vi "Basic Auton.vi"(1 "Auton RPM":dbl=4200.0, 2 "Auton Pitch":dbl=30.5) -> ()   [LabVIEW 2012]
uses:
  Robot Global Data.vi
panel:
  in  "stop log":bool
  in  "System Data On?":bool=TRUE
  in  "Sample?":bool=TRUE
  in  "Sample Rate (sec)":dbl=0.03
  out "Prime 3":i32
  out "Report 2":i32
  out "S3":i32
  out "Count 3":bool
  out "Prime 2.1":i32
  out "Prime 2":i32
  out "Report 1":i32
  out "S2":i32
  out "Count 2":bool
  out "Prime 1.1":i32
  out "Prime 1":i32
  out "S1":i32
  out "Count 1":bool
  # "Pre-Shot"
  # "Shoot 1"
  # "Shoot 2"
  # "Shoot 3"
  # "Was 0.1 at Palmetto"
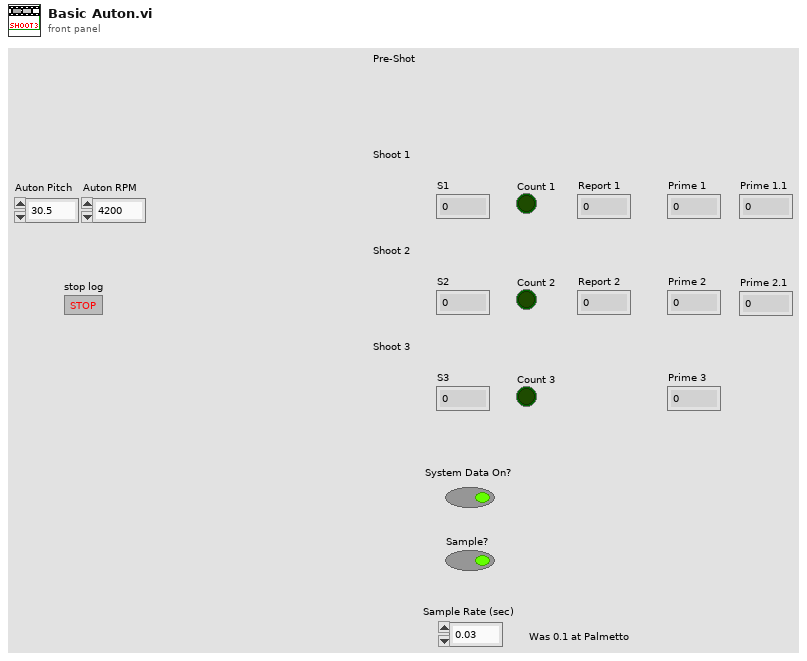
[diagram p1: front panel]
types:
  T1 = enum16{"open", "open or create", "create or replace", "create", "open (read-only)"}
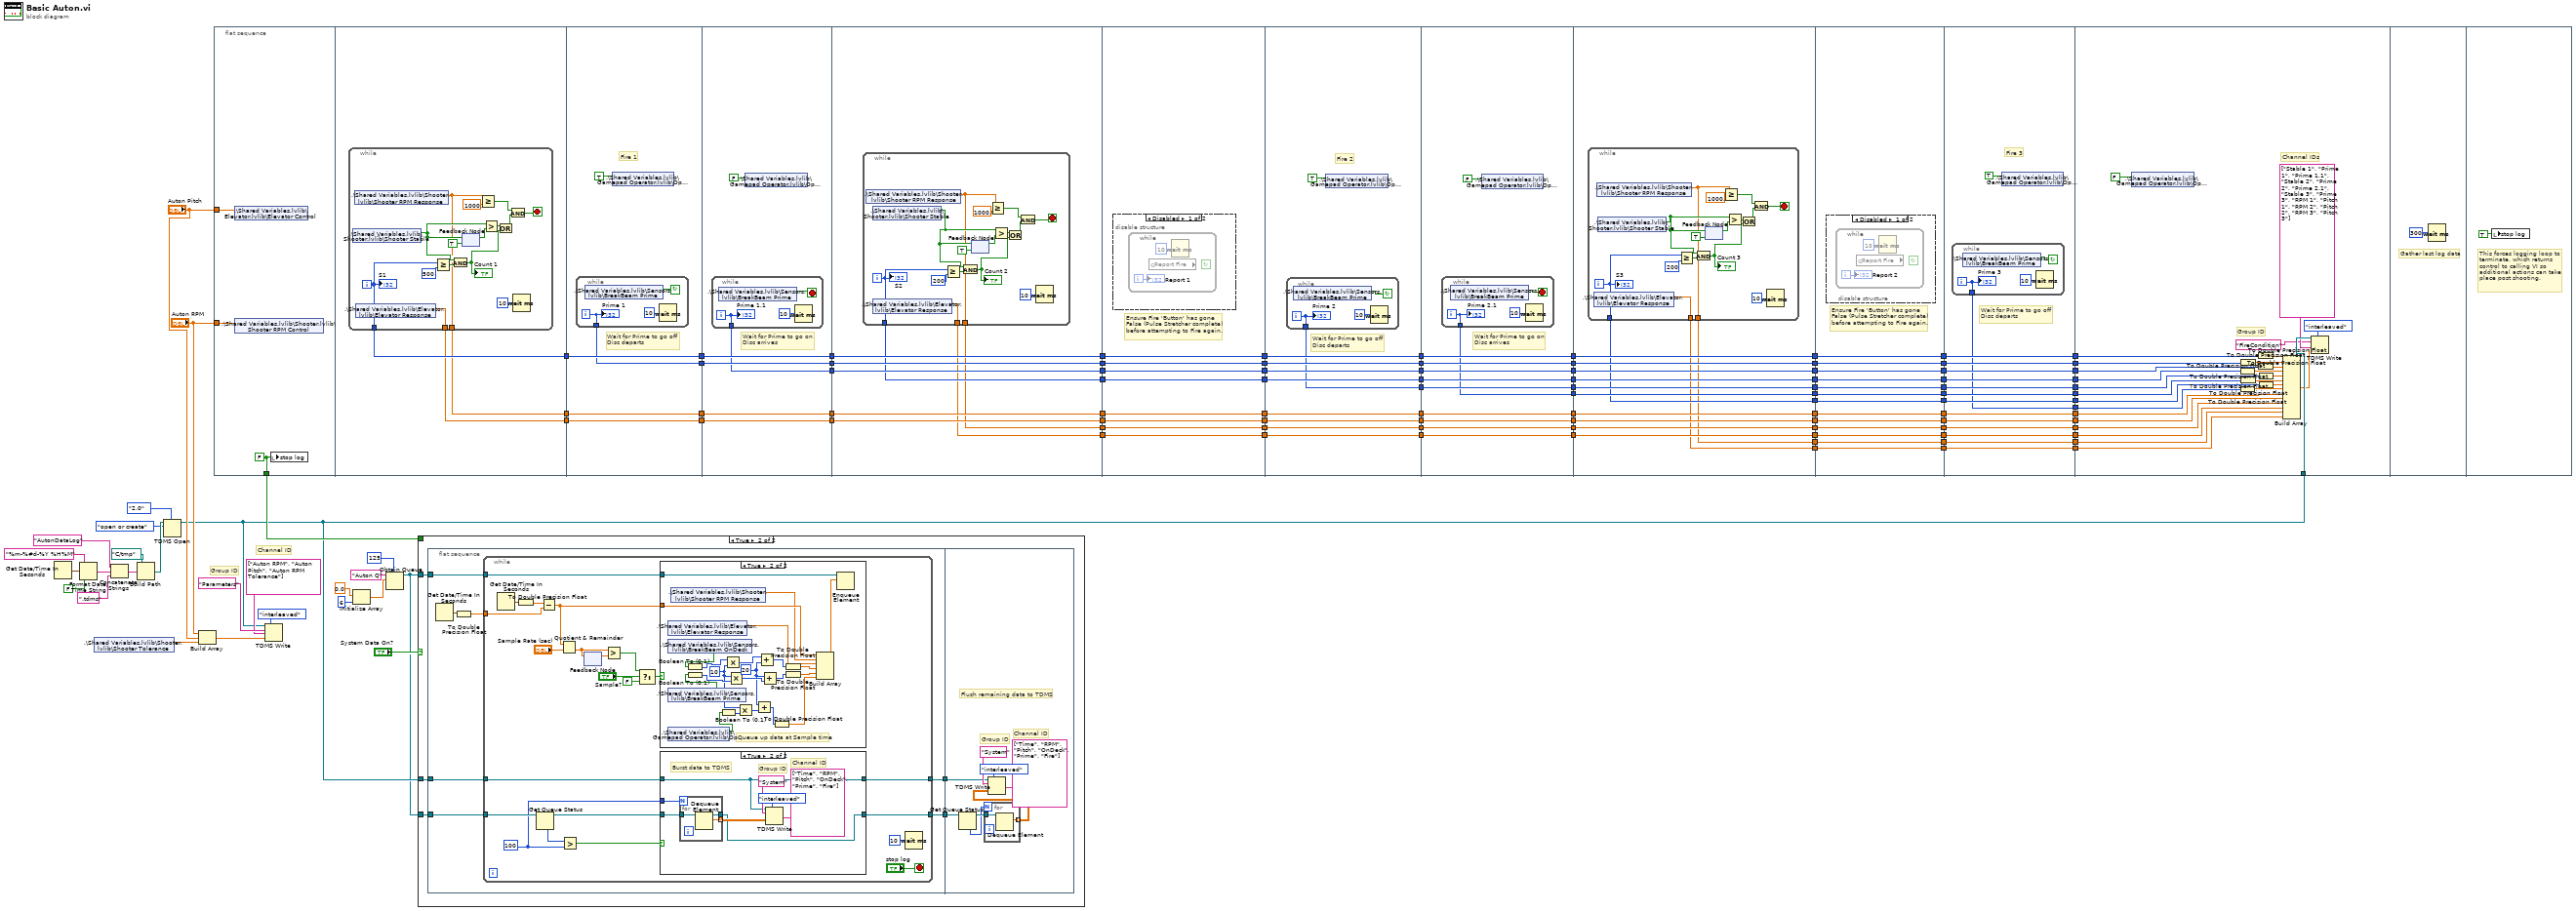
[diagram p0: block diagram]
diagram:
  # "Channel ID"
  # "Group ID"
  n1 = Get Date/Time In Seconds() -> (seconds since 1Jan1904=w17:timestamp)
  n2 = Format Date/Time String(time format string (%c)="%m-%#d-%Y %H%M", seconds (now)=w17, UTC format=FALSE) -> (date/time string=w22:string)
  n3 = shared-variable ".\\Shared Variables.lvlib\\Shooter.lvlib\\Shooter Tolerance"() -> (w10:dbl)  [unwired: 1 in, 1 out]
  n4 = Concatenate Strings("AutonDataLog" ("string"), w22, ".tdms" ("string")) -> (w24:string)
  n5 = Build Path(base path=path "C:/tmp" ("file path (dialog if empty)"), name or relative path=w24) -> (appended path=w25:path)
  n6 = TDMS Open(7:enum16{"1.0", "2.0"}."2.0" ("file format version (2.0)"), 10:T1."open or create" ("operation (0:open)"), 11:w25) -> (3:w7:refnum<k34>)  [unwired: 3 in, 1 out]
  n7 = Build Array("Auton RPM", "Auton Pitch", w10) -> (w13:dbl[])
  n8 = flat-sequence {
    tunnel: "Auton Pitch" -> [w116]
    tunnel: "Auton RPM" -> [w117]
    tunnel: [w115] -> w8
    tunnel: [w120] -> w114
    tunnel: [w119] -> w58
    tunnel: [w118] -> w48
    tunnel: w114 -> [w140]
    tunnel: [w140] -> w112
    tunnel: [w139] -> w96
    tunnel: [w138] -> w59
    tunnel: w58 -> [w138]
    tunnel: [w137] -> w49
    tunnel: w48 -> [w137]
    tunnel: [w149] -> w113
    tunnel: w112 -> [w149]
    tunnel: [w148] -> w97
    tunnel: w96 -> [w148]
    tunnel: [w147] -> w88
    tunnel: [w146] -> w60
    tunnel: w59 -> [w146]
    tunnel: [w145] -> w50
    tunnel: w49 -> [w145]
    tunnel: w113 -> [w160]
    tunnel: [w160] -> w108
    tunnel: [w159] -> w98
    tunnel: w97 -> [w159]
    tunnel: [w158] -> w89
    tunnel: w88 -> [w158]
    tunnel: [w157] -> w81
    tunnel: [w156] -> w61
    tunnel: w60 -> [w156]
    tunnel: [w155] -> w51
    tunnel: w50 -> [w155]
    tunnel: [w154] -> w41
    tunnel: [w153] -> w34
    tunnel: [w183] -> w109
    tunnel: w108 -> [w183]
    tunnel: [w182] -> w99
    tunnel: w98 -> [w182]
    tunnel: [w181] -> w90
    tunnel: w89 -> [w181]
    tunnel: [w180] -> w82
    tunnel: w81 -> [w180]
    tunnel: [w179] -> w62
    tunnel: w61 -> [w179]
    tunnel: [w178] -> w52
    tunnel: w51 -> [w178]
    tunnel: [w177] -> w42
    tunnel: w41 -> [w177]
    tunnel: [w176] -> w35
    tunnel: w34 -> [w176]
    tunnel: [w195] -> w110
    tunnel: w109 -> [w195]
    tunnel: [w194] -> w100
    tunnel: w99 -> [w194]
    tunnel: [w193] -> w91
    tunnel: w90 -> [w193]
    tunnel: [w192] -> w83
    tunnel: w82 -> [w192]
    tunnel: [w191] -> w76
    tunnel: [w190] -> w63
    tunnel: w62 -> [w190]
    tunnel: [w189] -> w53
    tunnel: w52 -> [w189]
    tunnel: [w188] -> w43
    tunnel: w42 -> [w188]
    tunnel: [w187] -> w36
    tunnel: w35 -> [w187]
    tunnel: [w209] -> w111
    tunnel: w110 -> [w209]
    tunnel: [w208] -> w101
    tunnel: w100 -> [w208]
    tunnel: [w207] -> w92
    tunnel: w91 -> [w207]
    tunnel: [w206] -> w84
    tunnel: w83 -> [w206]
    tunnel: [w205] -> w77
    tunnel: w76 -> [w205]
    tunnel: [w204] -> w72
    tunnel: [w203] -> w64
    tunnel: w63 -> [w203]
    tunnel: [w202] -> w54
    tunnel: w53 -> [w202]
    tunnel: [w201] -> w44
    tunnel: w43 -> [w201]
    tunnel: [w200] -> w37
    tunnel: w36 -> [w200]
    tunnel: w111 -> [w225]
    tunnel: [w225] -> w105
    tunnel: [w224] -> w102
    tunnel: w101 -> [w224]
    tunnel: [w223] -> w93
    tunnel: w92 -> [w223]
    tunnel: [w222] -> w85
    tunnel: w84 -> [w222]
    tunnel: [w221] -> w78
    tunnel: w77 -> [w221]
    tunnel: [w220] -> w73
    tunnel: w72 -> [w220]
    tunnel: [w219] -> w69
    tunnel: [w218] -> w65
    tunnel: w64 -> [w218]
    tunnel: [w217] -> w55
    tunnel: w54 -> [w217]
    tunnel: [w216] -> w45
    tunnel: w44 -> [w216]
    tunnel: [w215] -> w38
    tunnel: w37 -> [w215]
    tunnel: [w214] -> w31
    tunnel: [w213] -> w28
    tunnel: [w253] -> w106
    tunnel: w105 -> [w253]
    tunnel: [w252] -> w103
    tunnel: w102 -> [w252]
    tunnel: [w251] -> w94
    tunnel: w93 -> [w251]
    tunnel: [w250] -> w86
    tunnel: w85 -> [w250]
    tunnel: [w249] -> w79
    tunnel: w78 -> [w249]
    tunnel: [w248] -> w74
    tunnel: w73 -> [w248]
    tunnel: [w247] -> w70
    tunnel: w69 -> [w247]
    tunnel: [w246] -> w66
    tunnel: w65 -> [w246]
    tunnel: [w245] -> w56
    tunnel: w55 -> [w245]
    tunnel: [w244] -> w46
    tunnel: w45 -> [w244]
    tunnel: [w243] -> w39
    tunnel: w38 -> [w243]
    tunnel: [w242] -> w32
    tunnel: w31 -> [w242]
    tunnel: [w241] -> w29
    tunnel: w28 -> [w241]
    tunnel: [w270] -> w107
    tunnel: w106 -> [w270]
    tunnel: [w269] -> w104
    tunnel: w103 -> [w269]
    tunnel: [w268] -> w95
    tunnel: w94 -> [w268]
    tunnel: [w267] -> w87
    tunnel: w86 -> [w267]
    tunnel: [w266] -> w80
    tunnel: w79 -> [w266]
    tunnel: [w265] -> w75
    tunnel: w74 -> [w265]
    tunnel: [w264] -> w71
    tunnel: w70 -> [w264]
    tunnel: [w263] -> w68
    tunnel: [w262] -> w67
    tunnel: w66 -> [w262]
    tunnel: [w261] -> w57
    tunnel: w56 -> [w261]
    tunnel: [w260] -> w47
    tunnel: w46 -> [w260]
    tunnel: [w259] -> w40
    tunnel: w39 -> [w259]
    tunnel: [w258] -> w33
    tunnel: w32 -> [w258]
    tunnel: [w257] -> w30
    tunnel: w29 -> [w257]
    tunnel: w107 -> [w301]
    tunnel: w104 -> [w300]
    tunnel: w95 -> [w299]
    tunnel: w87 -> [w298]
    tunnel: w80 -> [w297]
    tunnel: w75 -> [w296]
    tunnel: w71 -> [w295]
    tunnel: w68 -> [w294]
    tunnel: w67 -> [w293]
    tunnel: w57 -> [w292]
    tunnel: w47 -> [w291]
    tunnel: w40 -> [w290]
    tunnel: w33 -> [w289]
    tunnel: w30 -> [w288]
    tunnel: w7 -> [w287]
    frame #0 {
      w115 = FALSE ("stop")
      n9 = shared-variable ".\\Shared Variables.lvlib\\Elevator.lvlib\\Elevator Control"(w116) -> ()  [unwired: 1 in, 1 out]
      n10 = shared-variable ".\\Shared Variables.lvlib\\Shooter.lvlib\\Shooter RPM Control"(w117) -> ()  [unwired: 1 in, 1 out]
      n11 = local write "stop log"(w115) -> ()
    }
    frame #1 {
      n12 = while {
        tunnel: [w124] -> w120
        tunnel: [w122] -> w119
        tunnel: [w121] -> w118
        i -> [w124]
        stop <- w125 stop-if-true
        n13 = shared-variable ".\\Shared Variables.lvlib\\Shooter.lvlib\\Shooter Stable"() -> (w123:bool)  [unwired: 1 in, 1 out]
        n14 = shared-variable ".\\Shared Variables.lvlib\\Shooter.lvlib\\Shooter RPM Response"() -> (w122:dbl)  [unwired: 1 in, 1 out]
        n15 = shared-variable ".\\Shared Variables.lvlib\\Elevator.lvlib\\Elevator Response"() -> (w121:dbl)  [unwired: 1 in, 1 out]
        n16 = Greater Or Equal?(x=w124, y=500) -> (x >= y?=w130:bool)
        n17 = And(x=w123, y=w130) -> (x .and. y?=w132:bool)
        "Count 1" <- w132
        n18 = feedback #1(TRUE ("Shooter Stable?")) -> (w128:bool)
        n19 = feedback-in #1(w123) -> ()
        n20 = Greater Or Equal?(x=w122, y=1000.0) -> (x >= y?=w127:bool)
        n21 = Greater?(x=w123, y=w128) -> (0:w133:bool)
        n22 = Or(x=w133, y=w132) -> (x .or. y?=w134:bool)
        n23 = And(x=w127, y=w134) -> (x .and. y?=w125:bool)
        n24 = Wait (ms)(milliseconds to wait=u32 10 ("millisecond multiple")) -> ()  [unwired: 1 out]
        "S1" <- w124
      }
    }
    frame #2 {
      # "Wait for Prime to go off\nDisc departs"
      # "Fire 1"
      n25 = while {
        tunnel: [w142] -> w139
        i -> [w142]
        stop <- w141 continue-if-true
        n26 = shared-variable ".\\Shared Variables.lvlib\\Sensors.lvlib\\BreakBeam Prime"() -> (w141:bool)  [unwired: 1 in, 1 out]
        n27 = Wait (ms)(milliseconds to wait=u32 10 ("millisecond multiple")) -> ()  [unwired: 1 out]
        "Prime 1" <- w142
      }
      n28 = shared-variable ".\\Shared Variables.lvlib\\Gamepad Operator.lvlib\\Op Button 6"(TRUE ("button5_Op")) -> ()  [unwired: 1 in, 1 out]
    }
    frame #3 {
      # "Wait for Prime to go on\nDisc arrives"
      n29 = while {
        tunnel: [w151] -> w147
        i -> [w151]
        stop <- w150 stop-if-true
        n30 = shared-variable ".\\Shared Variables.lvlib\\Sensors.lvlib\\BreakBeam Prime"() -> (w150:bool)  [unwired: 1 in, 1 out]
        n31 = Wait (ms)(milliseconds to wait=u32 10 ("millisecond multiple")) -> ()  [unwired: 1 out]
        "Prime 1.1" <- w151
      }
      n32 = shared-variable ".\\Shared Variables.lvlib\\Gamepad Operator.lvlib\\Op Button 6"(FALSE ("button5_Op")) -> ()  [unwired: 1 in, 1 out]
    }
    frame #4 {
      n33 = while {
        tunnel: [w164] -> w157
        tunnel: [w161] -> w154
        tunnel: [w162] -> w153
        i -> [w164]
        stop <- w165 stop-if-true
        n34 = shared-variable ".\\Shared Variables.lvlib\\Shooter.lvlib\\Shooter RPM Response"() -> (w161:dbl)  [unwired: 1 in, 1 out]
        n35 = shared-variable ".\\Shared Variables.lvlib\\Shooter.lvlib\\Shooter Stable"() -> (w163:bool)  [unwired: 1 in, 1 out]
        n36 = shared-variable ".\\Shared Variables.lvlib\\Elevator.lvlib\\Elevator Response"() -> (w162:dbl)  [unwired: 1 in, 1 out]
        n37 = Greater Or Equal?(x=w164, y=200) -> (x >= y?=w170:bool)
        n38 = And(x=w163, y=w170) -> (x .and. y?=w168:bool)
        "Count 2" <- w168
        n39 = feedback #2(TRUE ("Shooter Stable?")) -> (w172:bool)
        n40 = feedback-in #2(w163) -> ()
        n41 = Greater Or Equal?(x=w161, y=1000.0) -> (x >= y?=w173:bool)
        n42 = Greater?(x=w163, y=w172) -> (0:w167:bool)
        n43 = Or(x=w167, y=w168) -> (x .or. y?=w166:bool)
        n44 = And(x=w173, y=w166) -> (x .and. y?=w165:bool)
        n45 = Wait (ms)(milliseconds to wait=u32 10 ("millisecond multiple")) -> ()  [unwired: 1 out]
        "S2" <- w164
      }
    }
    frame #5 {
      # "Ensure Fire 'Button' has gone\nFalse (Pulse Stretcher complete)\nbefore attempting to Fire again."
      n46 = disable-structure shown="Disabled" {
        frame Disabled {
          n47 = while {
            i -> [w185]
            stop <- _ continue-if-true
            n48 = global read "Robot Global Data.vi" "Report Fire"() -> ()  [unwired: 1 out]
            n49 = Wait (ms)(milliseconds to wait=u32 10) -> ()  [unwired: 1 out]
            "Report 1" <- w185
          }
        }
        frame Enabled {
        }
      }
    }
    frame #6 {
      # "Wait for Prime to go off\nDisc departs"
      # "Fire 2"
      n50 = while {
        tunnel: [w197] -> w191
        i -> [w197]
        stop <- w196 continue-if-true
        n51 = shared-variable ".\\Shared Variables.lvlib\\Sensors.lvlib\\BreakBeam Prime"() -> (w196:bool)  [unwired: 1 in, 1 out]
        n52 = Wait (ms)(milliseconds to wait=u32 10 ("millisecond multiple")) -> ()  [unwired: 1 out]
        "Prime 2" <- w197
      }
      n53 = shared-variable ".\\Shared Variables.lvlib\\Gamepad Operator.lvlib\\Op Button 6"(TRUE ("button5_Op")) -> ()  [unwired: 1 in, 1 out]
    }
    frame #7 {
      # "Wait for Prime to go on\nDisc arrives"
      n54 = while {
        tunnel: [w211] -> w204
        i -> [w211]
        stop <- w210 stop-if-true
        n55 = shared-variable ".\\Shared Variables.lvlib\\Sensors.lvlib\\BreakBeam Prime"() -> (w210:bool)  [unwired: 1 in, 1 out]
        n56 = Wait (ms)(milliseconds to wait=u32 10 ("millisecond multiple")) -> ()  [unwired: 1 out]
        "Prime 2.1" <- w211
      }
      n57 = shared-variable ".\\Shared Variables.lvlib\\Gamepad Operator.lvlib\\Op Button 6"(FALSE ("button5_Op")) -> ()  [unwired: 1 in, 1 out]
    }
    frame #8 {
      n58 = while {
        tunnel: [w229] -> w219
        tunnel: [w226] -> w214
        tunnel: [w227] -> w213
        i -> [w229]
        stop <- w230 stop-if-true
        n59 = shared-variable ".\\Shared Variables.lvlib\\Elevator.lvlib\\Elevator Response"() -> (w227:dbl)  [unwired: 1 in, 1 out]
        n60 = shared-variable ".\\Shared Variables.lvlib\\Shooter.lvlib\\Shooter RPM Response"() -> (w226:dbl)  [unwired: 1 in, 1 out]
        n61 = shared-variable ".\\Shared Variables.lvlib\\Shooter.lvlib\\Shooter Stable"() -> (w228:bool)  [unwired: 1 in, 1 out]
        n62 = Greater Or Equal?(x=w229, y=200) -> (x >= y?=w235:bool)
        n63 = And(x=w228, y=w235) -> (x .and. y?=w237:bool)
        "Count 3" <- w237
        n64 = feedback #3(TRUE ("Shooter Stable?")) -> (w233:bool)
        n65 = feedback-in #3(w228) -> ()
        n66 = Greater Or Equal?(x=w226, y=1000.0) -> (x >= y?=w232:bool)
        n67 = Greater?(x=w228, y=w233) -> (0:w238:bool)
        n68 = Or(x=w238, y=w237) -> (x .or. y?=w239:bool)
        n69 = And(x=w232, y=w239) -> (x .and. y?=w230:bool)
        n70 = Wait (ms)(milliseconds to wait=u32 10 ("millisecond multiple")) -> ()  [unwired: 1 out]
        "S3" <- w229
      }
    }
    frame #9 {
      # "Ensure Fire 'Button' has gone\nFalse (Pulse Stretcher complete)\nbefore attempting to Fire again."
      n71 = disable-structure shown="Disabled" {
        frame Disabled {
          n72 = while {
            i -> [w255]
            stop <- _ continue-if-true
            n73 = global read "Robot Global Data.vi" "Report Fire"() -> ()  [unwired: 1 out]
            n74 = Wait (ms)(milliseconds to wait=u32 10) -> ()  [unwired: 1 out]
            "Report 2" <- w255
          }
        }
        frame Enabled {
        }
      }
    }
    frame #10 {
      # "Wait for Prime to go off\nDisc departs"
      # "Fire 3"
      n75 = while {
        tunnel: [w272] -> w263
        i -> [w272]
        stop <- w271 continue-if-true
        n76 = shared-variable ".\\Shared Variables.lvlib\\Sensors.lvlib\\BreakBeam Prime"() -> (w271:bool)  [unwired: 1 in, 1 out]
        n77 = Wait (ms)(milliseconds to wait=u32 10 ("millisecond multiple")) -> ()  [unwired: 1 out]
        "Prime 3" <- w272
      }
      n78 = shared-variable ".\\Shared Variables.lvlib\\Gamepad Operator.lvlib\\Op Button 6"(TRUE ("button5_Op")) -> ()  [unwired: 1 in, 1 out]
    }
    frame #11 {
      # "Channel IDs"
      # "Group ID"
      n79 = shared-variable ".\\Shared Variables.lvlib\\Gamepad Operator.lvlib\\Op Button 6"(FALSE ("button5_Op")) -> ()  [unwired: 1 in, 1 out]
      n80 = To Double Precision Float(number=w298) -> (double precision float=w278:dbl)
      n81 = To Double Precision Float(number=w294) -> (double precision float=w274:dbl)
      n82 = To Double Precision Float(number=w300) -> (double precision float=w282:dbl)
      n83 = To Double Precision Float(number=w296) -> (double precision float=w276:dbl)
      n84 = To Double Precision Float(number=w301) -> (double precision float=w280:dbl)
      n85 = To Double Precision Float(number=w299) -> (double precision float=w279:dbl)
      n86 = To Double Precision Float(number=w297) -> (double precision float=w277:dbl)
      n87 = To Double Precision Float(number=w295) -> (double precision float=w275:dbl)
      n88 = Build Array(w280, w282, w279, w278, w277, w276, w275, w274, w293, w292, w291, w290, w289, w288) -> (w283:dbl[])
      n89 = TDMS Write(0:w287, 1:enum16{"decimated", "interleaved"}."interleaved" ("data layout (0:decimated)"), 5:"FireCondition" ("group name in (Untitled)"), 7:string[] ["Stable 1", "Prime 1", "Prime 1.1", "Stable 2", "Prime 2", "Prime 2.1", "Stable 3", "Prime 3", "RPM 1", "Pitch 1", "RPM 2", "Pitch 2", "RPM 3", "Pitch 3"] ("channel name(s) in (Untitled)"), 9:w283) -> ()  [unwired: 1 in, 4 out]
    }
    frame #12 {
      # "Gather last log data"
      n90 = Wait (ms)(milliseconds to wait=u32 300) -> ()  [unwired: 1 out]
    }
    frame #13 {
      # "This forces logging loop to\nterminate, which returns \ncontrol to calling VI so \nadditional actions can take \nplace post shooting."
      n91 = local write "stop log"(TRUE ("stop")) -> ()
    }
  }
  n92 = TDMS Write(0:w7, 1:enum16{"decimated", "interleaved"}."interleaved" ("data layout (0:decimated)"), 5:"Parameters" ("group name in (Untitled)"), 7:string[] ["Auton RPM", "Auton Pitch", "Auton RPM Tolerance"] ("channel name(s) in (Untitled)"), 9:w13) -> ()  [unwired: 1 in, 4 out]
  n93 = Initialize Array(0.0, 6 ("dimension size")) -> (w2:dbl[])
  n94 = Obtain Queue(max queue size (-1, unlimited)=125, name (unnamed)="Auton Q", element data type=w2) -> (queue out=w1:refnum<queue>)  [unwired: 2 in, 2 out]
  n95 = case shown="True" "System Data On?" {
    tunnel: w8 -> [_ _]
    tunnel: w7 -> [_ w308]
    tunnel: w1 -> [_ w307]
    tunnel: w1 -> [_ w306]
    frame False {
    }
    frame True {
      n96 = flat-sequence {
        tunnel: w308 -> [w313]
        tunnel: w307 -> [w312]
        tunnel: w306 -> [w311]
        tunnel: [w310] -> w305
        tunnel: [w309] -> w304
        tunnel: w305 -> [w376]
        tunnel: w304 -> [w377]
        frame #0 {
          n97 = Get Date/Time In Seconds() -> (seconds since 1Jan1904=w315:timestamp)
          n98 = To Double Precision Float(number=w315) -> (double precision float=w314:dbl)
          n99 = while {
            tunnel: w314 -> [w329]
            tunnel: w313 -> [w324]
            tunnel: w312 -> [w323]
            tunnel: w311 -> [w322]
            tunnel: [w318] -> w310
            tunnel: [w317] -> w309
            stop <- "stop log" stop-if-true
            w316 = 100 ("y")
            n100 = Get Date/Time In Seconds() -> (seconds since 1Jan1904=w333:timestamp)
            n101 = To Double Precision Float(number=w333) -> (double precision float=w332:dbl)
            n102 = Get Queue Status(queue=w322) -> (queue out=w321:refnum<queue>, # elements in queue=w319:i32)  [unwired: 2 in, 6 out]
            n103 = Subtract(x=w332, y=w329) -> (x-y=w326:dbl)
            n104 = Quotient & Remainder(x=w326, y="Sample Rate (sec)") -> (floor(x/y)=w330:dbl)  [unwired: 1 out]
            n105 = Greater?(x=w319, y=w316) -> (0:w320:bool)
            n106 = feedback #4() -> (w331:dbl)  [unwired: 1 in]
            n107 = feedback-in #4(w330) -> ()
            n108 = Greater?(x=w330, y=w331) -> (0:w327:bool)
            n109 = Select(t=w327, s="Sample?", f=FALSE) -> (s? t:f=w335:bool)
            n110 = case shown="True" w335 {
              tunnel: w326 -> [_ w372]
              tunnel: w323 -> [_ w352]
              frame False {
                # "Logging is Off"
              }
              frame True {
                w362 = 10 ("y")
                w360 = i16 20 ("y")
                # "Queue up data at Sample time"
                n111 = shared-variable ".\\Shared Variables.lvlib\\Elevator.lvlib\\Elevator Response"() -> (w355:dbl)  [unwired: 1 in, 1 out]
                n112 = shared-variable ".\\Shared Variables.lvlib\\Sensors.lvlib\\BreakBeam OnDeck"() -> (w353:bool)  [unwired: 1 in, 1 out]
                n113 = shared-variable ".\\Shared Variables.lvlib\\Sensors.lvlib\\BreakBeam Prime"() -> (w354:bool)  [unwired: 1 in, 1 out]
                n114 = shared-variable ".\\Shared Variables.lvlib\\Gamepad Operator.lvlib\\Op Button 6"() -> (w357:bool)  [unwired: 1 in, 1 out]
                n115 = shared-variable ".\\Shared Variables.lvlib\\Shooter.lvlib\\Shooter RPM Response"() -> (w356:dbl)  [unwired: 1 in, 1 out]
                n116 = Boolean To (0,1)(Boolean=w353) -> (0, 1=w369:i16)
                n117 = Boolean To (0,1)(Boolean=w354) -> (0, 1=w368:i16)
                n118 = Boolean To (0,1)(Boolean=w357) -> (0, 1=w363:i16)
                n119 = Multiply(x=w369, y=w362) -> (x*y=w367:i32)
                n120 = Multiply(x=w362, y=w368) -> (x*y=w366:i32)
                n121 = Multiply(x=w362, y=w363) -> (x*y=w361:i32)
                n122 = Add(x=w360, y=w361) -> (x+y=w359:i32)
                n123 = Add(x=w367, y=w360) -> (x+y=w365:i32)
                n124 = Add(x=w360, y=w366) -> (x+y=w364:i32)
                n125 = To Double Precision Float(number=w359) -> (double precision float=w358:dbl)
                n126 = To Double Precision Float(number=w365) -> (double precision float=w371:dbl)
                n127 = To Double Precision Float(number=w364) -> (double precision float=w370:dbl)
                n128 = Build Array(w372, w356, w355, w371, w370, w358) -> (w351:dbl[])
                n129 = Enqueue Element(queue=w352, element=w351) -> ()  [unwired: 2 in, 3 out]
              }
            }
            n130 = case shown="True" w320 {
              tunnel: w324 -> [w338 w340]
              tunnel: w321 -> [w339 w345]
              tunnel: w316 -> [_ w342]
              tunnel: [w339 w341] -> w318
              tunnel: [w338 w340] -> w317
              frame False {
              }
              frame True {
                # "Burst data to TDMS"
                # "Channel ID"
                # "Group ID"
                n131 = for {
                  N: w342 -> [_]
                  tunnel: [w350] -> w346 mode=indexing
                  tunnel: w345 -> [w349]
                  tunnel: [w348] -> w341
                  n132 = Dequeue Element(queue=w349) -> (queue out=w348:refnum<queue>, element=w350:dbl[])  [unwired: 2 in, 2 out]
                }
                n133 = TDMS Write(0:w340, 1:enum16{"decimated", "interleaved"}."interleaved" ("data layout (0:decimated)"), 5:"System" ("group name in (Untitled)"), 7:string[] ["Time", "RPM", "Pitch", "OnDeck", "Prime", "Fire"] ("channel name(s) in (Untitled)"), 9:w346) -> ()  [unwired: 1 in, 4 out]
              }
            }
            n134 = Wait (ms)(milliseconds to wait=u32 10) -> ()  [unwired: 1 out]
          }
        }
        frame #1 {
          # "Flush remaining data to TDMS"
          # "Channel ID"
          # "Group ID"
          n135 = Get Queue Status(queue=w376) -> (queue out=w375:refnum<queue>, # elements in queue=w374:i32)  [unwired: 2 in, 6 out]
          n136 = for {
            N: w374 -> [_]
            tunnel: w375 -> [w382]
            tunnel: [w381] -> w373 mode=indexing
            n137 = Dequeue Element(queue=w382) -> (element=w381:dbl[])  [unwired: 2 in, 3 out]
          }
          n138 = TDMS Write(0:w377, 1:enum16{"decimated", "interleaved"}."interleaved" ("data layout (0:decimated)"), 5:"System" ("group name in (Untitled)"), 7:string[] ["Time", "RPM", "Pitch", "OnDeck", "Prime", "Fire"] ("channel name(s) in (Untitled)"), 9:w373) -> ()  [unwired: 1 in, 4 out]
        }
      }
    }
  }
